vi "usrp get tx antenna.vi"(7 "strbuffer_len":u64, 8 "error in (no error)":errorcluster, 9 "ant_out":string, 10 "chan":u64, 11 "h":u64) -> (0 "error out":errorcluster, 1 "ant_out out":string, 2 "function return":u32(ring), 3 "h 2":u64)   [LabVIEW 2024, in "uhd.lvlib"]
doc: "UHD_API uhd_error uhd_usrp_get_tx_antenna(\n uhd_usrp_handle h, size_t chan, char* ant_out, size_t strbuffer_len);"
uses:
  uhd.lvlib
  uhd.so
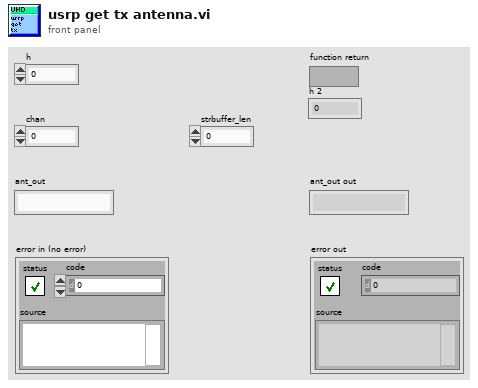
[diagram p1: front panel]
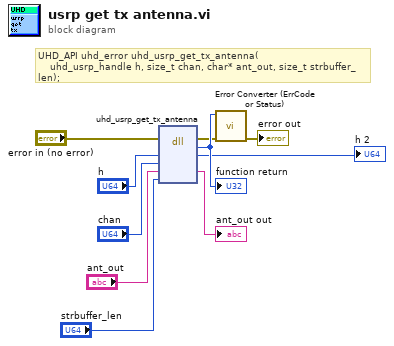
[diagram p0: block diagram]
diagram:
  # "UHD_API uhd_error uhd_usrp_get_tx_antenna(\n    uhd_usrp_handle h, size_t chan, char* ant_out, size_t strbuffer_len);"
  n1 = dll-call lib="uhd.*" fn="uhd_usrp_get_tx_antenna"(error in="error in (no error)", "h"="h", "chan"="chan", "ant_out"="ant_out", "strbuffer_len"="strbuffer_len") -> (error out=w3:errorcluster, w10:u32, "h"=→"h 2":u64, "ant_out"=→"ant_out out":string)  [unwired: 4 in, 1 out]
  "function return" <- w10
  n2 = call "Error Converter (ErrCode or Status).vi"("error in (no error)"=w3, "error code"=w10) -> ("error out"=→"error out":errorcluster)  [unwired: 9 in]
